vi "Do.vi"(8 "error in (no error)":errorcluster, 9 "Events":refnum<class "Events.lvclass">, 10 "Message Loop Data in":T1, 11 "Yield JSON in":refnum<class "Yield JSON.lvclass">) -> (0 "error out":errorcluster, 1 "Write request":T9, 2 "Message Loop Data out":T1, 3 "Yield JSON out":refnum<class "Yield JSON.lvclass">)   [LabVIEW 2020, in "wamplv.lvlib" / "Yield JSON.lvclass"]
uses:
  Yield JSON.lvclass
  Yield JSON.lvclass/Yield JSON.ctl
  Utils/Utils.lvclass
  wamplv.lvlib
  42cd12d4-b0be-47c8-ab9e-f4aa5ff4b0df.vi
  TypeDefs/WAMP Message Codes.ctl
  WAMP Client/Private/TypeDef/Publish Requests Map.ctl
  WAMP Client/Private/TypeDef/Endpoint Data.ctl
  Call/ICallRequest/ICallRequest.lvclass
  WAMP Client/Private/TypeDef/CALL Request Map.ctl
  WAMP Client/Private/TypeDef/SUBSCRIBE Requests Map.ctl
  WAMP Client/Private/TypeDef/Subscriptions Map.ctl
  WAMP Client/Private/TypeDef/Unsubscribe Requests Map.ctl
  WAMP Client/Private/TypeDef/Unregister requests map.ctl
  WAMP Client/Private/TypeDef/Message Loop Data.ctl
  TypeDefs/Transport type.ctl
  WAMP Client/Private/TypeDef/Write queue item.ctl
  Events/EventsParent/Events.lvclass
  Subscribe/ISubscribe/ISubscribe.lvclass
  Publish/IPublish/IPublish.lvclass
  Message loop classes/Subscription details/SubscriptionDetailsParent/SubscriptionDetailsParent.lvclass
  Unsubscribe/IUnsubscribe/IUnsubscribe.lvclass
  Register/IRegister/IRegister.lvclass
  Unregister/IUnregister/IUnregister.lvclass
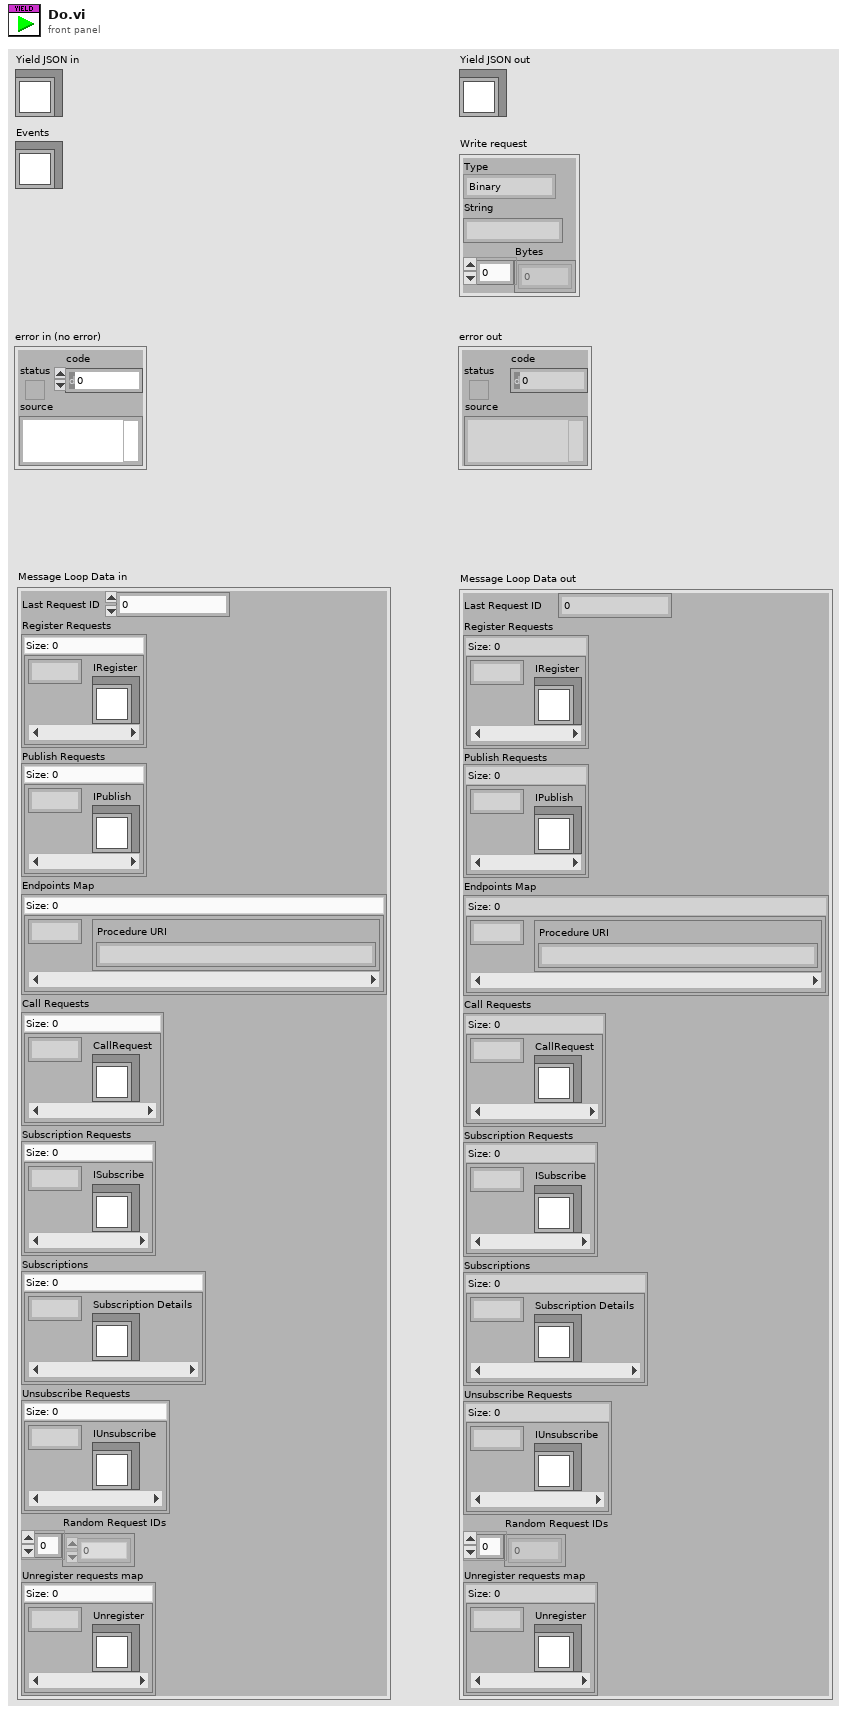
[diagram p1: front panel]
types:
  T1 = typedef "wamplv.lvlib/Message Loop Data.ctl" = cluster{"Last Request ID":u64, "Register Requests":map{u64, refnum<class "IRegister.lvclass">}, "Publish Requests":T2, "Endpoints Map":map{u64, T3}, "Call Requests":T4, "Subscription Requests":T5, "Subscriptions":T6, "Unsubscribe Requests":T7, "Random Request IDs":u64[], "Unregister requests map":T8}
  T2 = typedef "wamplv.lvlib/Publish Requests Map.ctl" = map{u64, refnum<class "IPublish.lvclass">}
  T3 = typedef "wamplv.lvlib/Endpoint Data.ctl" = cluster{"Procedure URI":string}
  T4 = typedef "wamplv.lvlib/CALL Request Map.ctl" = map{u64, refnum<class "ICallRequest.lvclass">}
  T5 = typedef "wamplv.lvlib/SUBSCRIBE Requests Map.ctl" = map{u64, refnum<class "ISubscribe.lvclass">}
  T6 = typedef "wamplv.lvlib/Subscriptions Map.ctl" = map{u64, refnum<class "SubscriptionDetailsParent.lvclass">}
  T7 = typedef "wamplv.lvlib/Unsubscribe Requests Map.ctl" = map{u64, refnum<class "IUnsubscribe.lvclass">}
  T8 = typedef "wamplv.lvlib/Unregister requests map.ctl" = map{u64, refnum<class "IUnregister.lvclass">}
  T9 = typedef "wamplv.lvlib/Write queue item.ctl" = cluster{"Type":T10, "String":string, "Bytes":u8[]}
  T10 = typedef "wamplv.lvlib/Transport type.ctl" = enum16{"Binary", "Text"}
  T11 = typedef "wamplv.lvlib/WAMP Message Codes.ctl" = enum8{"HELLO", "WELCOME", "CHALLENGE", "AUTHENTICATE", "ABORT", "GOODBYE", "ERROR", "PUBLISH", "PUBLISHED", "SUBSCRIBE", "SUBSCRIBED", "UNSUBSCRIBE", "UNSUBSCRIBED", "EVENT", "CALL", "RESULT", "REGISTER", "REGISTERED", "UNREGISTER", "UNREGISTERED", "INVOCATION", "YIELD"}
  T12 = typedef "wamplv.lvlib/YIELD request data (JSON).ctl" = cluster{"Invocation Request ID":u64, "Arguments":string, "ArgumentsKw":string, "Options":string}
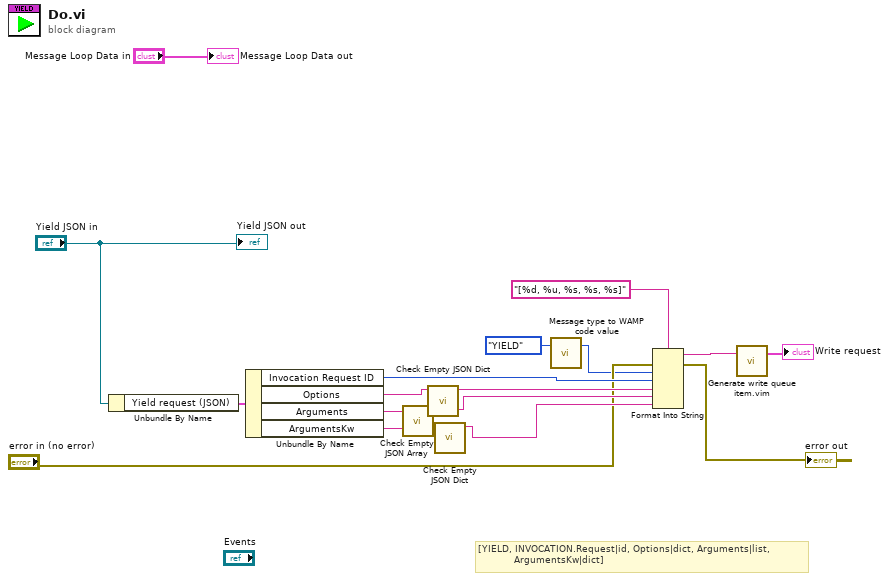
[diagram p0: block diagram]
diagram:
  # "[YIELD, INVOCATION.Request|id, Options|dict, Arguments|list,\n            ArgumentsKw|dict]"
  n1 = Unbundle By Name("Yield JSON in") -> ("Yield request (JSON)"=w2:T12)
  n2 = Unbundle By Name(w2) -> ("Invocation Request ID"=w11:u64, "Options"=w14:string, "Arguments"=w17:string, "ArgumentsKw"=w12:string)
  n3 = call "Check Empty JSON Array.vi"("JSON in"=w17) -> ("JSON out"=w16:string)  [unwired: 10 in]
  n4 = call "Check Empty JSON Dict.vi"("JSON in"=w14) -> ("JSON out"=w15:string)  [unwired: 10 in]
  n5 = call "Check Empty JSON Dict.vi"("JSON in"=w12) -> ("JSON out"=w13:string)  [unwired: 10 in]
  n6 = call "Message type to WAMP code value.vi"("Message Type"=WAMP_Message_Codes."YIELD") -> ("WAMP Numeric value"=w5:u8)  [unwired: 2 in]
  n7 = Format Into String(format string="[%d, %u, %s, %s, %s]" ("element"), error in="error in (no error)", w5, w11, w15, w16, w13) -> (resulting string=w7:string, error out=→"error out":errorcluster)  [unwired: 1 in]
  n8 = call "Generate write queue item.vim"("Input"=w7) -> ("Ouput"=→"Write request":T9)  [unwired: 2 in]
  "Yield JSON out" <- "Yield JSON in"
  "Message Loop Data out" <- "Message Loop Data in"
